vi "Init_core.vi"(8 "error in (no error)":errorcluster, 10 "VIRefIn":refnum<vi>, 11 "ctlrRef_VAT in":refnum<class "ctlRef_VAT.lvclass">) -> (0 "error out":errorcluster, 3 "ctlrRef_VAT out":refnum<class "ctlRef_VAT.lvclass">)   [LabVIEW 2020, in "CtlReferences.lvlib" / "ctlRef_VAT.lvclass"]
uses:
  ctlRef_VAT.lvclass
  ctlRef_VAT.lvclass/ctlRef_VAT.ctl
  CtlReferences/CtlReferences.lvclass
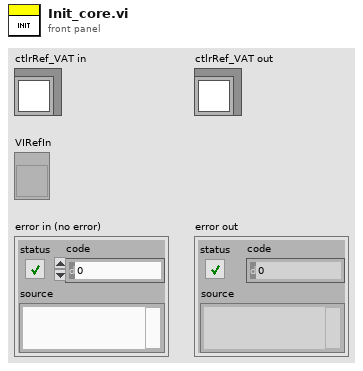
[diagram p1: front panel]
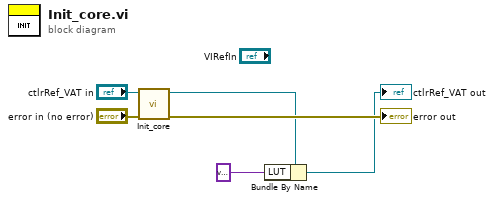
[diagram p0: block diagram]
diagram:
  n1 = call-parent "Init_core.vi"("error in (no error)"="error in (no error)", "CtlReferences in"="ctlrRef_VAT in") -> ("error out"=→"error out":errorcluster, "CtlReferences out"=w2:refnum<class "ctlRef_VAT.lvclass">)  [unwired: 8 in]
  n2 = Bundle By Name(cluster=w2, "LUT"=variant ("ControlVariant")) -> (→"ctlrRef_VAT out":refnum<class "ctlRef_VAT.lvclass">)
